vi "Show Data Logger.vi"(8 "error in":errorcluster, 11 "Series Actor in":refnum<class "Series Actor.lvclass">) -> (0 "error out":errorcluster, 3 "Series Actor out":refnum<class "Series Actor.lvclass">)   [LabVIEW 2023, in "Series Actor.lvlib" / "Series Actor.lvclass"]
uses:
  Series Actor.lvclass
  Series Actor.lvclass/Series Actor.ctl
  <vilib>/MGI/Panel Manager/Panel Actor/Panel Actor Messages/Show Panel Msg/Show Panel Msg.lvclass
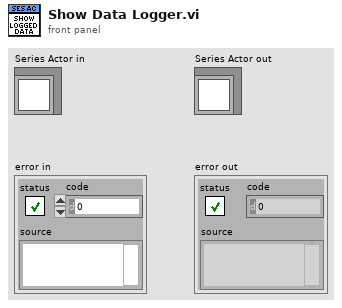
[diagram p1: front panel]
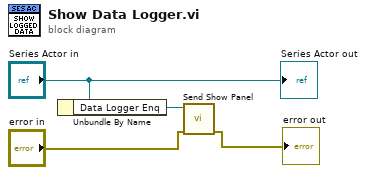
[diagram p0: block diagram]
diagram:
  n1 = Unbundle By Name("Series Actor in") -> ("Data Logger Enq"=w3:refnum<class "Message Enqueuer.lvclass">)
  n2 = call <vilib>:"Send Show Panel.vi"("Error In"="error in", "Message Enqueuer in"=w3) -> ("Error Out"=→"error out":errorcluster)  [unwired: 8 in, 1 out]
  "Series Actor out" <- "Series Actor in"
